vi "Read FPGA Reference.vi"(8 "error in (no error)":errorcluster, 11 "System Modules Factory in":refnum<class "System Modules Factory.lvclass">) -> (0 "error out":errorcluster, 2 "FPGA Reference.lvclass":refnum<class "FPGA Reference.lvclass">, 3 "System Modules Factory out":refnum<class "System Modules Factory.lvclass">)   [LabVIEW 2019, in "System Modules Factory.lvclass"]
uses:
  System Modules Factory.lvclass
  SPIM Library/Hardware Actors/Parents/FPGA Reference/FPGA Reference.lvclass
  System Modules Factory.lvclass/System Modules Factory.ctl
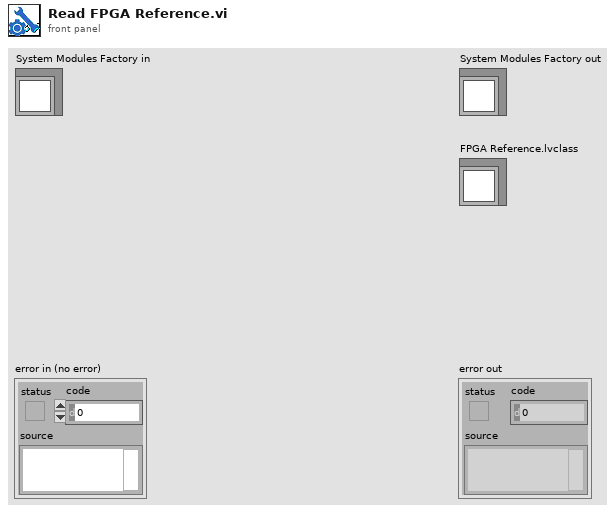
[diagram p1: front panel]
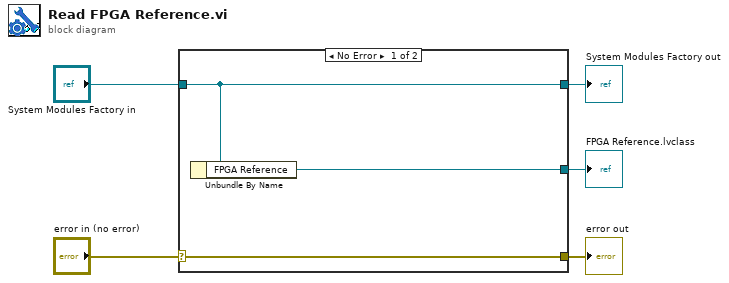
[diagram p0: block diagram]
diagram:
  n1 = case shown="No Error" "error in (no error)" {
    selector: "error in (no error)" -> [w8 w9]
    tunnel: [w8 w9] -> w4
    tunnel: [w7 w10] -> w2
    tunnel: "System Modules Factory in" -> [w7 w10]
    tunnel: [w6 _] -> w1
    frame No Error {
      n2 = Unbundle By Name(w7) -> ("FPGA Reference"=w6:refnum<class "FPGA Reference.lvclass">)
    }
    frame Error {
    }
  }
  "error out" <- w4
  "System Modules Factory out" <- w2
  "FPGA Reference.lvclass" <- w1
